vi "Private_NumberOfGcodeConfig.vi"(8 "error in (no error)":errorcluster, 11 "XuLyStringUART in":refnum<class "XuLyStringUART.lvclass">) -> (0 "error out":errorcluster, 2 "McodeConfigNumber":dbl, 3 "XuLyStringUART out":refnum<class "XuLyStringUART.lvclass">)   [LabVIEW 2014, in "LibraryGcode.lvlib" / "XuLyStringUART.lvclass"]
uses:
  XuLyStringUART.lvclass
  XuLyStringUART.lvclass/XuLyStringUART.ctl
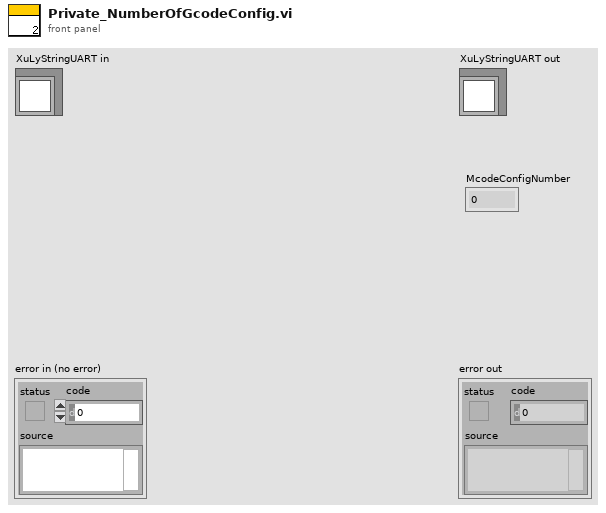
[diagram p1: front panel]
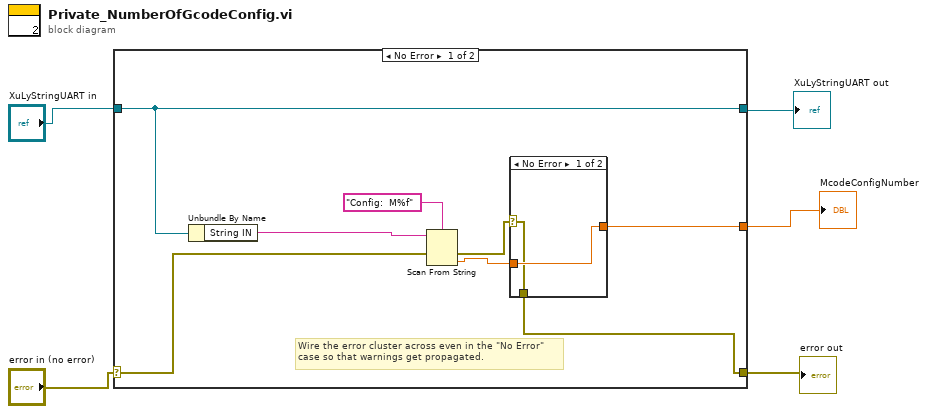
[diagram p0: block diagram]
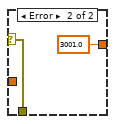
[diagram p2: hidden frame]
diagram:
  n1 = case shown="No Error" "error in (no error)" {
    selector: "error in (no error)" -> [w10 w19]
    tunnel: [w8 w19] -> w3
    tunnel: [w7 w18] -> w4
    tunnel: "XuLyStringUART in" -> [w7 w18]
    tunnel: [w11 _] -> w1
    frame No Error {
      # "Wire the error cluster across even in the \"No Error\"\ncase so that warnings get propagated."
      n2 = Unbundle By Name(w7) -> ("String IN"=w6:string)
      n3 = Scan From String(format string="Config:  M%f", input string=w6, error in=w10) -> (error out=w9:errorcluster, output 1=w12:dbl)  [unwired: 2 in, 2 out]
      n4 = case shown="No Error" w9 {
        selector: w9 -> [w14 w16]
        tunnel: [w15 3001.0] -> w11
        tunnel: w12 -> [w15 _]
        tunnel: [w14 w16] -> w8
        frame No Error {
        }
        frame Error {
        }
      }
    }
    frame Error {
    }
  }
  "error out" <- w3
  "XuLyStringUART out" <- w4
  "McodeConfigNumber" <- w1
